vi "Segment Log File.vi"(8 "error in (no error)":errorcluster, 11 "Segmented Log in":refnum<class "Segmented Log.lvclass">) -> (0 "error out":errorcluster, 2 "Segment Log File":bool, 3 "Segmented Log out":refnum<class "Segmented Log.lvclass">)   [LabVIEW 2012, in "Waveform Data Logger Engine.lvlib" / "Segmented Log.lvclass"]
doc: "Checks whether a given condition has been met that indicates the current log file instance should be closed."
uses:
  Segmented Log.lvclass
  Segmented Log.lvclass/Segmented Log.ctl
  Footprint Segmented Log/Footprint Segmented Log.lvclass
  Footprint Segmented Log/Footprint Segmented Log.lvclass/Footprint Segmented Log.ctl
  Log Files/Log File/Log File.lvclass/Log File.ctl
  Time Segmented Log/Time Segmented Log.lvclass
  Get Current Log File Instance.vi
  Log Files/Log File/Get File Size.vi
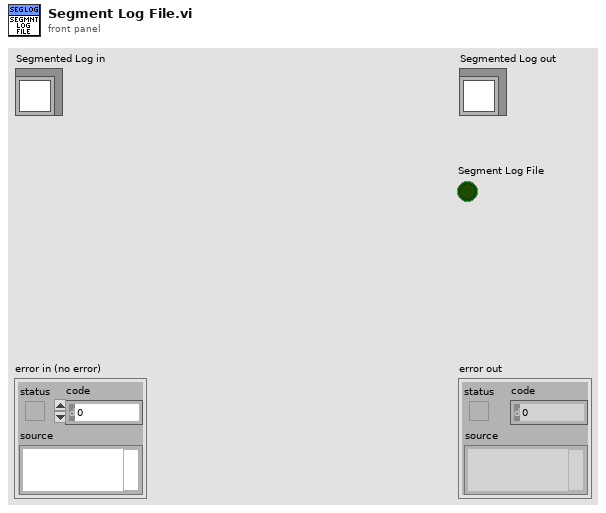
[diagram p1: front panel]
types:
  T1 = typedef "Waveform Data Logger Engine.lvlib/Segmented Log.lvclass/Segmented Log Type.ctl" = enum16{"No Limit", "Footprint", "Time"}
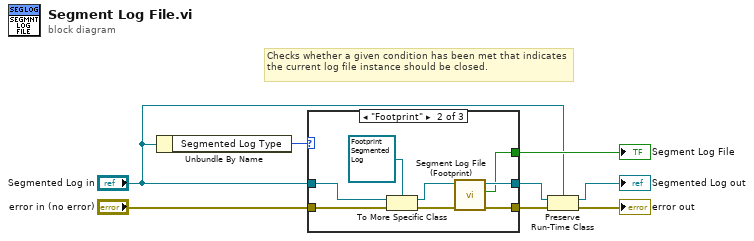
[diagram p0: block diagram]
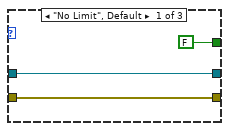
[diagram p2: hidden frame]
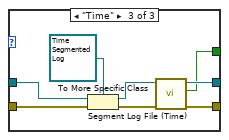
[diagram p3: hidden frame]
diagram:
  # "Checks whether a given condition has been met that indicates the current log file instance should be closed."
  n1 = Unbundle By Name("Segmented Log in") -> ("Segmented Log Type"=w8:T1)
  n2 = case shown="\"Footprint\"" w8 {
    tunnel: "Segmented Log in" -> [w11 w17 w25]
    tunnel: "error in (no error)" -> [w10 w19 w27]
    tunnel: [w11 w14 w22] -> w2
    tunnel: [w10 w13 w21] -> w5
    tunnel: [FALSE ("Segment Log File") w12 w20] -> w6
    frame "No Limit", Default {
    }
    frame "Footprint" {
      n3 = To More Specific Class(target class=refnum<class "Footprint Segmented Log.lvclass"> refnum ("Footprint Segmented Log.lvclass"), reference=w17, error in=w19) -> (specific class reference=w15:refnum<class "Footprint Segmented Log.lvclass">, error out=w18:errorcluster)
      n4 = call "Segment Log File (Footprint).vi"("error in (no error)"=w18, "Footprint Segmented Log in"=w15) -> ("error out"=w13:errorcluster, "Segment Log File"=w12:bool, "Footprint Segmented Log out"=w14:refnum<class "Footprint Segmented Log.lvclass">)  [unwired: 7 in]
    }
    frame "Time" {
      n5 = To More Specific Class(target class=refnum<class "Time Segmented Log.lvclass"> refnum ("Time Segmented Log.lvclass"), reference=w25, error in=w27) -> (specific class reference=w23:refnum<class "Time Segmented Log.lvclass">, error out=w26:errorcluster)
      n6 = call "Segment Log File (Time).vi"("error in (no error)"=w26, "Time Segmented Log in"=w23) -> ("error out"=w21:errorcluster, "Segment Log File"=w20:bool, "Time Segmented Log out"=w22:refnum<class "Time Segmented Log.lvclass">)  [unwired: 7 in]
    }
  }
  "Segment Log File" <- w6
  n7 = Preserve Run-Time Class(object in=w2, error in=w5, 2:"Segmented Log in") -> (object out=→"Segmented Log out":refnum<class "Segmented Log.lvclass">, error out=→"error out":errorcluster)
